vi "TwoEdge.vi"() -> ()   [LabVIEW 2015]
doc: "This VI performs a two edge separation measurement between PB1 and PB2. It outputs the difference in milliseconds between rising edges of PB1 and PB2.\n\nLED0 on the sbRIO evaluation board is illuminated after PB1 is pushed. LED0 and LED1 is illuminated after PB2 is pushed."
uses:
  <vilib>/Platform/TimedLoop/XDataNode/timing_clust.ctl
  <vilib>/Platform/TimedLoop/XDataNode/nitl_modes.ctl
  <vilib>/Platform/TimedLoop/XDataNode/wakeup.ctl
  <vilib>/rvi/Emulation/niFpgaSctlEmulationGetInTimedLoop.vi
  <vilib>/rvi/Emulation/niFpgaEmulationReportErrorSimple.vi
  <vilib>/rvi/Emulation/niFpgaGetClockAttributes.vi
  <vilib>/rvi/Emulation/niFpgaCriticalErrorInLSC.vi
  <vilib>/rvi/eio/common/nirviEmuTemplateMethod_errors.vi
  <vilib>/Platform/TimedLoop/XDataNode/XDataNode.xnode
  <vilib>/eio/EIONode/EIONode.xnode
  <vilib>/Platform/TimedLoop/XDataNode/XDNodeRunTimeDep.lvlib
panel:
  in  "stop":bool
  out "Separation (ms)":u32
  # "This VI performs a two edge separation measurement \nbetween PB1 and PB2.  It outputs the difference in \nmilliseconds between rising edges of PB1 and PB2.\n\nLED0 on the LabVIEW RIO evaluation board is illuminated \nafter PB1 is pushed.  LED0 and LED1 is illuminated after PB2 \nis pushed."
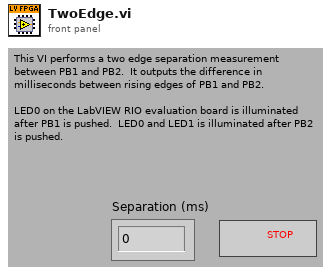
[diagram p1: front panel]
types:
  T1 = typedef "XDNodeRunTimeDep.lvlib/timing_clust.ctl" = cluster{"Expected End [f-1]":u64, "Actual End [f-1]":u64, "Finished Late? [f-1]":bool, "Expected End [i-1]":u64, "Actual End [i-1]":u64, "Finished Late? [i-1]":bool, "Expected Start [i]":u64, "Actual Start [i]":u64, "Expected Start [f]":u64, "Actual Start [f]":u64, "Source Name":string, "Structure Name":string, "Period":i64, "Deadline":i64, "Offset":i64, "Start":i64, "Priority":i32, "Timeout":i32, "Mode":T2, "Wakeup Reason":T3, "Error":errorcluster, "Source Type":string, "Secondary Source Type":string, "Global End Time":u64, "Global Start Time":u64, "Frame Duration":u64, "Iteration Duration":u64, "Assigned CPU":i32, "I/O Scan Engine Mode":u32}
  T2 = typedef "XDNodeRunTimeDep.lvlib/nitl_modes.ctl" = enum32{"No Change", "Process missed periods, maintain original phase", "Discard missed periods, maintain original phase", "Process missed periods, ignore original phase", "Discard missed periods, ignore original phase"}
  T3 = typedef "XDNodeRunTimeDep.lvlib/wakeup.ctl" = enum32{"Normal", "Aborted", "Asynchronous wakeup", "Timing source error", "Timed loop error", "Timeout"}
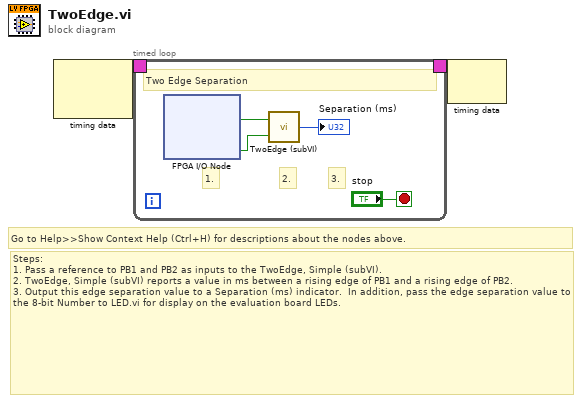
[diagram p0: block diagram]
diagram:
  # "Go to Help>>Show Context Help (Ctrl+H) for descriptions about the nodes above."
  # "Steps:\n1. Pass a reference to PB1 and PB2 as inputs to the TwoEdge, Simple (subVI).\n2. TwoEdge, Simple (subVI) reports a value in ms between a rising edge of PB1 and a rising edge of PB2.\n3. Output this edge separation value to a Separation (ms) indicator.  In addition, pass the edge separation value to the 8-bit Number to LED.vi for display on the evaluation board LEDs."
  n1 = node-c288() -> (w1:T1)  [unwired: 2 out]
  n2 = timed-loop {
    timing-out: [_] -> w2
    timing: w1 -> [_]
    stop <- "stop" stop-if-true
    # "3."
    # "2."
    # "1."
    # "Two Edge Separation"
    n3 = xnode "FPGA I/O Node"() -> ("PB1"=w5:bool, "PB2"=w3:bool)  [unwired: 2 in, 2 out]
    n4 = call "TwoEdge (subVI).vi"("Input 1"=w3, "Input 0"=w5) -> ("Edge Separation (ms)"=→"Separation (ms)":u32)
  }
  n5 = node-c288(w2) -> ()  [unwired: 1 out]
